vi "email report.vi"() -> ()   [LabVIEW 2019]
panel:
  in  "notification interval (min)":dbl
  in  "notify\nprocess\nstart?":bool
  in  "process":T1(ring)
  in  "stop":bool
  in  "To":string
  out "XY Graph":cluster{dbl[], dbl[]}[](graph)
  # "use semicolon (;) for multiple receipents"
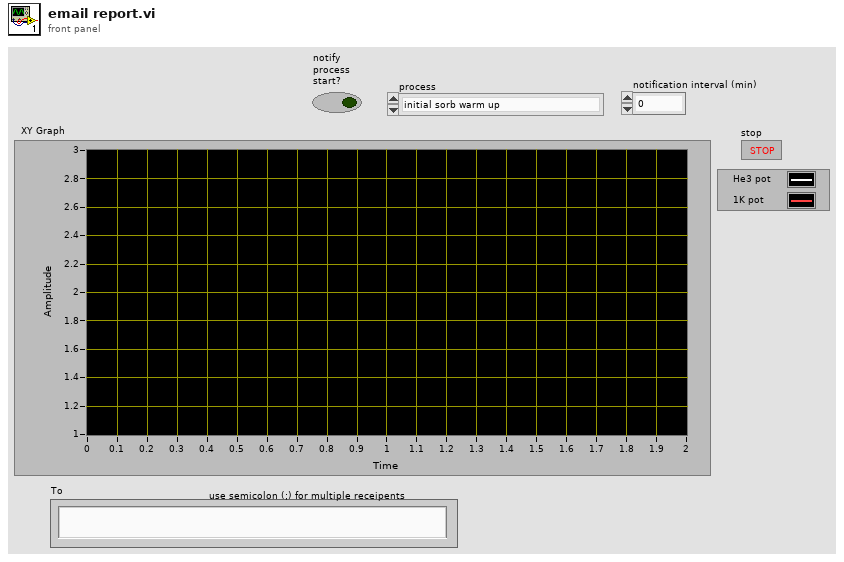
[diagram p1: front panel]
types:
  T1 = enum16{"initial sorb warm up", "condensation stage"}
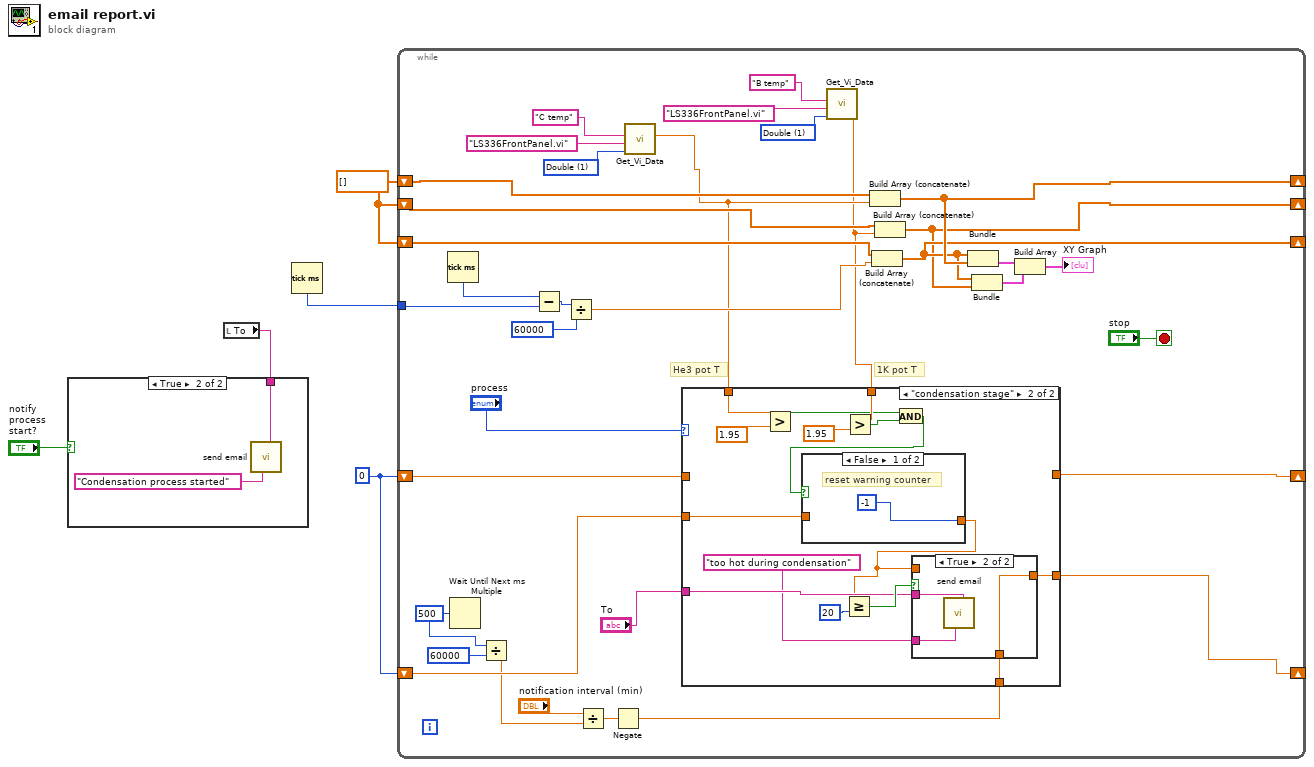
[diagram p0: block diagram]
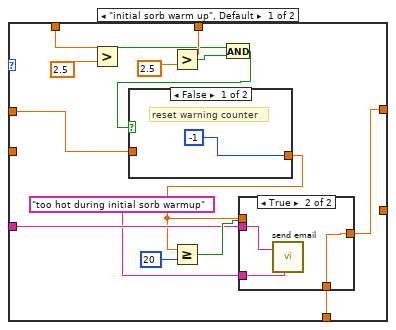
[diagram p3: hidden frame]
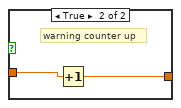
[diagram p5: hidden frame]
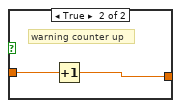
[diagram p7: hidden frame]
diagram:
  w1 = 0
  w4 = dbl[] []
  n1 = local read "To"() -> (w2:string)
  n2 = case shown="True" "notify\nprocess\nstart?" {
    tunnel: w2 -> [_ w6]
    frame False {
    }
    frame True {
      n3 = call "send email.vi"("To"=w6, "Subject"="Condensation process started") -> ()  [unwired: 10 in]
    }
  }
  n4 = Tick Count (ms)() -> (millisecond timer value=w5:u32)
  n5 = while {
    tunnel: w5 -> [w35]
    shift-right: [w28] -> _
    shift-left: w4 -> [w32]
    shift-right: [w26] -> _
    shift-left: w4 -> [w31]
    shift-right: [w27] -> _
    shift-left: w4 -> [w30]
    shift-right: [w17] -> _
    shift-left: w1 -> [w18]
    shift-right: [w14] -> _
    shift-left: w1 -> [w15]
    stop <- "stop" stop-if-true
    w13 = u32 500 ("millisecond multiple")
    w37 = u16 1 items=["String", "Double", "Boolean", "Variant"] ("Data Type")
    w40 = u16 1 items=["String", "Double", "Boolean", "Variant"] ("Data Type")
    # "1K pot T"
    # "He3 pot T"
    n6 = Tick Count (ms)() -> (millisecond timer value=w36:u32)
    n7 = Wait Until Next ms Multiple(millisecond multiple=w13) -> ()  [unwired: 1 out]
    n8 = Divide(x=w13, y=u32 60000) -> (x/y=w10:dbl)
    n9 = Subtract(x=w36, y=w35) -> (x-y=w34:u32)
    n10 = Divide(x=w34, y=u32 60000) -> (x/y=w29:dbl)
    n11 = Divide(x="notification interval (min)", y=w10) -> (x/y=w9:dbl)
    n12 = Negate(x=w9) -> (-x=w8:dbl)
    n13 = call "Get_Vi_Data.vi"("Data Type"=w40, "VI name"="LS336FrontPanel.vi" ("Control Name"), "Control Name"="C temp") -> ("Data (Double)"=w20:dbl)  [unwired: 4 in, 4 out]
    n14 = call "Get_Vi_Data.vi"("Data Type"=w37, "VI name"="LS336FrontPanel.vi" ("Control Name"), "Control Name"="B temp") -> ("Data (Double)"=w19:dbl)  [unwired: 4 in, 4 out]
    n15 = case shown="\"condensation stage\"" "process" {
      tunnel: w20 -> [w57 w79]
      tunnel: w19 -> [w55 w77]
      tunnel: w18 -> [w50 _]
      tunnel: [w45 _] -> w17
      tunnel: "To" -> [w47 w70]
      tunnel: w15 -> [_ w67]
      tunnel: [_ w66] -> w14
      tunnel: w8 -> [w43 w65]
      frame "initial sorb warm up", Default {
        n16 = Greater?(x=w57, y=2.5) -> (0:w53:bool)
        n17 = Greater?(x=w55, y=2.5) -> (0:w52:bool)
        n18 = And(x=w53, y=w52) -> (x .and. y?=w51:bool)
        n19 = case shown="False" w51 {
          tunnel: [-1 w64] -> w44
          tunnel: w50 -> [_ w63]
          frame False {
            # "reset warning counter"
          }
          frame True {
            # "warning counter up"
            n20 = Increment(x=w63) -> (x+1=w64:dbl)
          }
        }
        n21 = Greater Or Equal?(x=w44, y=20) -> (x >= y?=w48:bool)
        n22 = case shown="True" w48 {
          tunnel: w47 -> [_ w61]
          tunnel: "too hot during initial sorb warmup" -> [_ w60]
          tunnel: [w58 w59] -> w45
          tunnel: w44 -> [w58 _]
          tunnel: w43 -> [_ w59]
          frame False {
          }
          frame True {
            n23 = call "send email.vi"("To"=w61, "Subject"=w60) -> ()  [unwired: 10 in]
          }
        }
      }
      frame "condensation stage" {
        n24 = Greater?(x=w79, y=1.95) -> (0:w75:bool)
        n25 = Greater?(x=w77, y=1.95) -> (0:w74:bool)
        n26 = And(x=w75, y=w74) -> (x .and. y?=w73:bool)
        n27 = case shown="False" w73 {
          tunnel: [-1 w86] -> w68
          tunnel: w67 -> [_ w85]
          frame False {
            # "reset warning counter"
          }
          frame True {
            # "warning counter up"
            n28 = Increment(x=w85) -> (x+1=w86:dbl)
          }
        }
        n29 = Greater Or Equal?(x=w68, y=20) -> (x >= y?=w71:bool)
        n30 = case shown="True" w71 {
          tunnel: w70 -> [_ w83]
          tunnel: "too hot during condensation" -> [_ w82]
          tunnel: [w80 w81] -> w66
          tunnel: w68 -> [w80 _]
          tunnel: w65 -> [_ w81]
          frame False {
          }
          frame True {
            n31 = call "send email.vi"("To"=w83, "Subject"=w82) -> ()  [unwired: 10 in]
          }
        }
      }
    }
    n32 = Build Array (concatenate)(w32, w20) -> (w28:dbl[])
    n33 = Build Array (concatenate)(w30, w29) -> (w27:dbl[])
    n34 = Build Array (concatenate)(w31, w19) -> (w26:dbl[])
    n35 = Bundle(w27, w28) -> (w25:cluster{dbl[], dbl[]})  [unwired: 1 in]
    n36 = Bundle(w27, w26) -> (w24:cluster{dbl[], dbl[]})  [unwired: 1 in]
    n37 = Build Array(w25, w24) -> (→"XY Graph":cluster{dbl[], dbl[]}[])
  }
